vi "Select Channels.vi"(8 "error in (no error)":errorcluster, 11 "Node Ptr":u64 format="%.0x") -> (0 "error out":errorcluster)   [LabVIEW 2023, in "Protection and Counter Addon System Explorer.lvlib"]
uses:
  Protection and Counter Addon System Explorer.lvlib
  Addon Shared/SubVIs/GUID Lookup.vi
  SubModules/Frame-Protection-Support/Source/System Explorer/Protection and Counter Support System Explorer.lvlib
  Addon Shared/Protection and Counter Addon Shared.lvlib
panel:
  in  "Tag":string
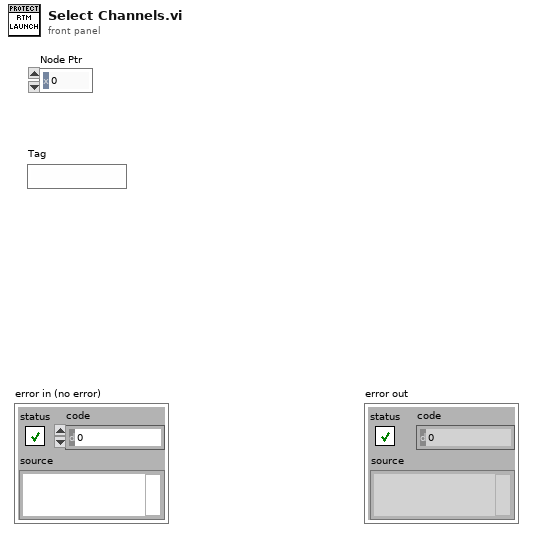
[diagram p1: front panel]
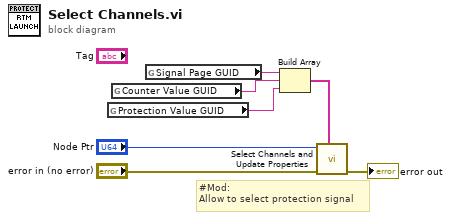
[diagram p0: block diagram]
diagram:
  # "#Mod:\nAllow to select protection signal"
  n1 = global read "GUID Lookup.vi" "Protection Value GUID"() -> (w1:string)
  n2 = global read "GUID Lookup.vi" "Counter Value GUID"() -> (w4:string)
  n3 = global read "GUID Lookup.vi" "Signal Page GUID"() -> (w3:string)
  n4 = Build Array(w3, w4, w1) -> (w2:string[])
  n5 = call "Select Channels and Update Properties.vi"("guids"=w2, "error in (no error)"="error in (no error)", "Node Ptr"="Node Ptr") -> ("error out"=→"error out":errorcluster)  [unwired: 8 in]
